vi "Subscribe.vi"(8 "error in (no error)":errorcluster, 10 "Key":string="myhome/kitchen/temp", 11 "Zenoh in":refnum<class "Zenoh.lvclass">) -> (0 "error out":errorcluster, 3 "Zenoh out":refnum<class "Zenoh.lvclass">)   [LabVIEW 2021, in "Zenoh.lvclass"]
doc: "Create a subscription to a specific key. Once subscribed updated values to that key will be stored and can be polled by reader VIs. A handle to the key is created in a map. The reader will look up the handle using the key."
uses:
  Zenoh.lvclass
  Zenoh.lvclass/Zenoh.ctl
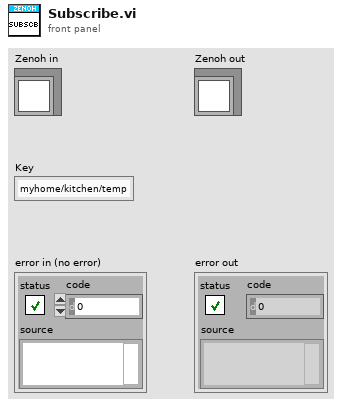
[diagram p1: front panel]
types:
  T1 = typedef "Zenoh.lvclass/Channel Info.ctl" = cluster{"Mime Type":string, "Reader Handle":u64}
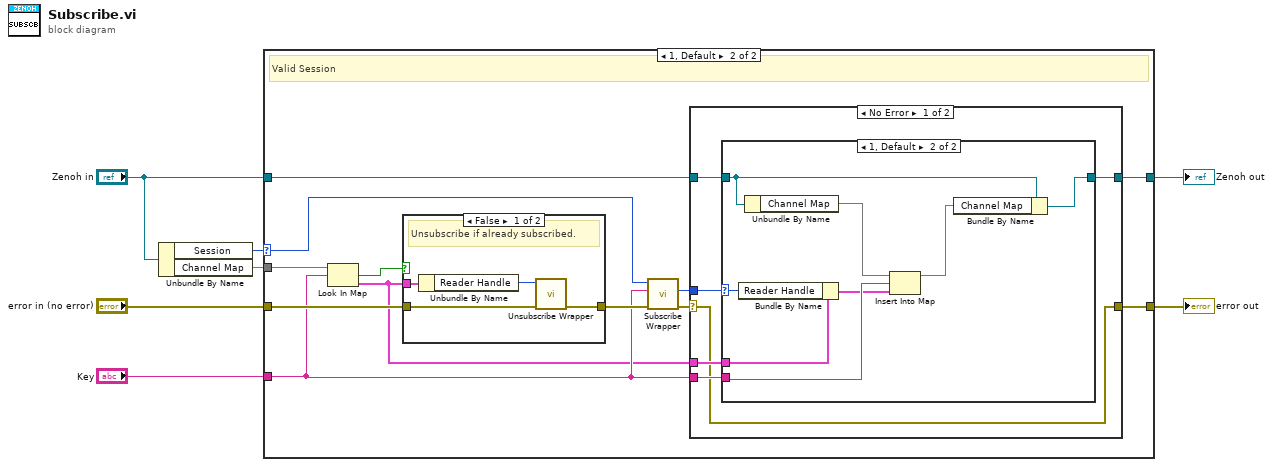
[diagram p0: block diagram]
diagram:
  n1 = Unbundle By Name("Zenoh in") -> ("Session"=w3:u64, "Channel Map"=w4:map{string, T1})
  n2 = case shown="1, Default" w3 {
    selector: w3 -> [_ w20]
    tunnel: "Key" -> [_ w14]
    tunnel: "error in (no error)" -> [w8 w21]
    tunnel: "Zenoh in" -> [w9 w15]
    tunnel: w4 -> [_ w18]
    tunnel: [w8 w11] -> w2
    tunnel: [w9 w10] -> w1
    frame 0 {
      # "Invalid session"
    }
    frame 1, Default {
      # "Valid Session"
      n3 = Look In Map(map=w18, key=w14) -> (key not found?=w17:bool, value=w13:T1)  [unwired: 1 in]
      n4 = case shown="False" w17 {
        tunnel: w21 -> [w42 w43]
        tunnel: w13 -> [w41 _]
        tunnel: [w39 w43] -> w19
        frame False {
          # "Unsubscribe if already subscribed."
          n5 = Unbundle By Name(w41) -> ("Reader Handle"=w40:u64)
          n6 = call "Unsubscribe Wrapper.vi"("error in (no error)"=w42, "Reader Handle"=w40) -> ("error out"=w39:errorcluster)  [unwired: 9 in]
        }
        frame True {
        }
      }
      n7 = call "Subscribe Wrapper.vi"("error in (no error)"=w19, "key"=w14, "Session in"=w20) -> ("error out"=w12:errorcluster, "Reader Handle"=w16:u64)  [unwired: 7 in]
      n8 = case shown="No Error" w12 {
        selector: w12 -> [w22 w37]
        tunnel: w16 -> [w27 _]
        tunnel: w15 -> [w26 w38]
        tunnel: w14 -> [w25 _]
        tunnel: w13 -> [w24 _]
        tunnel: [w23 w38] -> w10
        tunnel: [w22 w37] -> w11
        frame No Error {
          n9 = case shown="1, Default" w27 {
            selector: w27 -> [_ w33]
            tunnel: w26 -> [w28 w31]
            tunnel: w25 -> [_ w35]
            tunnel: w24 -> [_ w34]
            tunnel: [w28 w29] -> w23
            frame 0 {
            }
            frame 1, Default {
              n10 = Bundle By Name(cluster=w34, "Reader Handle"=w33) -> (w32:T1)
              n11 = Unbundle By Name(w31) -> ("Channel Map"=w36:map{string, T1})
              n12 = Insert Into Map(map in=w36, key=w35, value=w32) -> (map out=w30:map{string, T1})  [unwired: 2 out]
              n13 = Bundle By Name(cluster=w31, "Channel Map"=w30) -> (w29:refnum<class "Zenoh.lvclass">)
            }
          }
        }
        frame Error {
        }
      }
    }
  }
  "error out" <- w2
  "Zenoh out" <- w1
